vi "SeCrTs-AO Start .vi"(8 "error in":errorcluster, 9 "AO config":T1(array[cluster]), 11 "Refnum in":refnum<k21>) -> (0 "error out":errorcluster, 3 "Refnum out":refnum<k21>)   [LabVIEW 2022 SP3]
doc: "This VI is for start for Analog Output"
uses:
  <vilib>/DAQmx/configure/timing.llb/DAQmx Timing (Sample Clock).vi
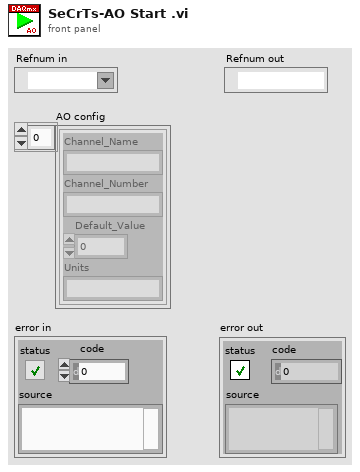
[diagram p1: front panel]
types:
  T1 = cluster{"Channel_Name":string, "Channel_Number":string, "Default_Value":dbl, "Units":string}[]
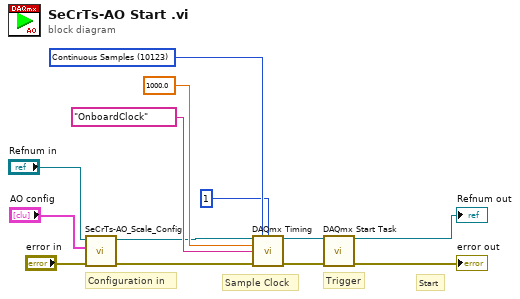
[diagram p0: block diagram]
diagram:
  w9 = 10123 items=["Finite Samples"=10178, "Continuous Samples"=10123, "Hardware Timed Single Point"=12522] ("sample mode")
  # "Start"
  # "Trigger"
  # "Sample Clock"
  # "Configuration in"
  n1 = call "SeCrTs-AO_Scale_Config.vi"("error in (no error)"="error in", "AO config"="AO config", "Refnum in"="Refnum in") -> ("error out"=w6:errorcluster, "Refnum out"=w5:refnum<k21>)  [unwired: 7 in]
  n2 = call-poly <vilib>:"DAQmx Timing.vi"("task/channels in"=w5, "sample mode"=w9, "samples per channel"=1, "rate"=1000.0, "source"=tag "OnboardClock", "error in"=w6) -> ("task out"=w12:refnum<k21>, "error out"=w7:errorcluster)  [unwired: 8 in]
  n3 = call <vilib>:"DAQmx Start Task.vi"("task/channels in"=w12, "error in"=w7) -> ("task out"=→"Refnum out":refnum<k21>, "error out"=→"error out":errorcluster)  [unwired: 12 in]
